vi "XP2i_Check_Error.vi"(4 "Error Code":T6=5490, 6 "Driver Name":T7="B1_28", 8 "Error In":errorcluster, 11 "DriverConnect in":T1={"InterfaceType"=enum."VISA", "OpenedSession"="COM4", "InterfaceSettings"={"Interface"=enum."RS232", "EOS 4 read"=enum."Default (=EOS 4 write)", "EOS 4 write"=enum."CR (\\r)", "TMO, ms"=2000, "Sett"=variant(cluster{"Baud Rate":u32, "Data Bits":u16, "Parity":u16, "Stop Bits":u16, "Flow Control":u16, "Eho":bool} {"Baud Rate"=75, "Data Bits"=0, "Parity"=0, "Stop Bits"=0, "Flow Control"=0, "Eho"=FALSE})}}) -> (0 "Error Out":errorcluster, 3 "DriverConnect out":T1={"InterfaceType"=enum."VISA", "OpenedSession"="COM4", "InterfaceSettings"={"Interface"=enum."RS232", "EOS 4 read"=enum."Default (=EOS 4 write)", "EOS 4 write"=enum."CR (\\r)", "TMO, ms"=2000, "Sett"=variant(cluster{"Baud Rate":u32, "Data Bits":u16, "Parity":u16, "Stop Bits":u16, "Flow Control":u16, "Eho":bool} {"Baud Rate"=75, "Data Bits"=0, "Parity"=0, "Stop Bits"=0, "Flow Control"=0, "Eho"=FALSE})}})   [LabVIEW 2018]
uses:
  MOKO_LabViewLibrary/MokoLowLevel/MokoLowLovelControl/MLLC_DriverName.ctl
  MOKO_LabViewLibrary/MokoLowLevel/MokoLowLovelControl/MLLC_ErrorCode.ctl
  MOKO_LabViewLibrary/MokoLowLevel/MokoLowLovelControl/MLLC_ConnectCluster.ctl
  MOKO_LabViewLibrary/MokoLowLevel/MokoLowLovelControl/MLLC_InterfaceType.ctl
  MOKO_LabViewLibrary/MokoLowLevel/MokoLowLovelControl/MLLC_OpenedSession.ctl
  MOKO_LabViewLibrary/MokoLowLevel/MokoLowLovelControl/MLLC_InterfaceSettings.ctl
  MOKO_LabViewLibrary/MokoLowLevel/MokoLowLovelControl/MLLC_InterfaceKind.ctl
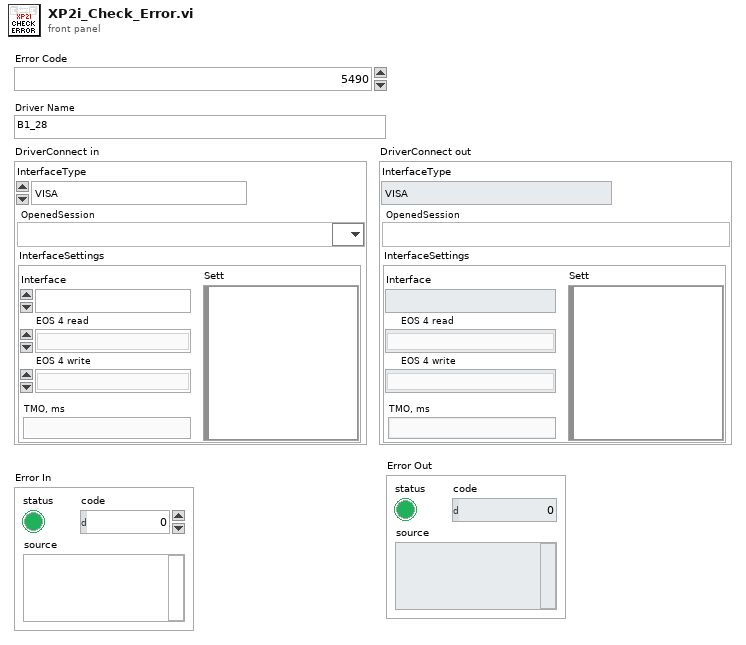
[diagram p1: front panel]
types:
  T1 = typedef "MLLC_ConnectCluster.ctl" = cluster{"InterfaceType":T2, "OpenedSession":T3, "InterfaceSettings":T4}
  T2 = typedef "MLLC_InterfaceType.ctl" = enum16{"VISA", "Prologix USB-GPIB"}
  T3 = typedef "MLLC_OpenedSession.ctl" = refnum<visa-resource-name>
  T4 = typedef "MLLC_InterfaceSettings.ctl" = cluster{"Interface":T5, "EOS 4 read":enum16{"Default (=EOS 4 write)", "CR (\\r)", "LF (\\n)", "None"}, "EOS 4 write":enum16{"CR+LF (\\r\\n)", "CR (\\r)", "LF (\\n)", "None"}, "TMO, ms":i32, "Sett":variant}
  T5 = typedef "MLLC_InterfaceKind.ctl" = enum16{"RS232", "GPIB", "USB", "Ethernet", "another"}
  T6 = typedef "MLLC_ErrorCode.ctl" = u32
  T7 = typedef "MLLC_DriverName.ctl" = string
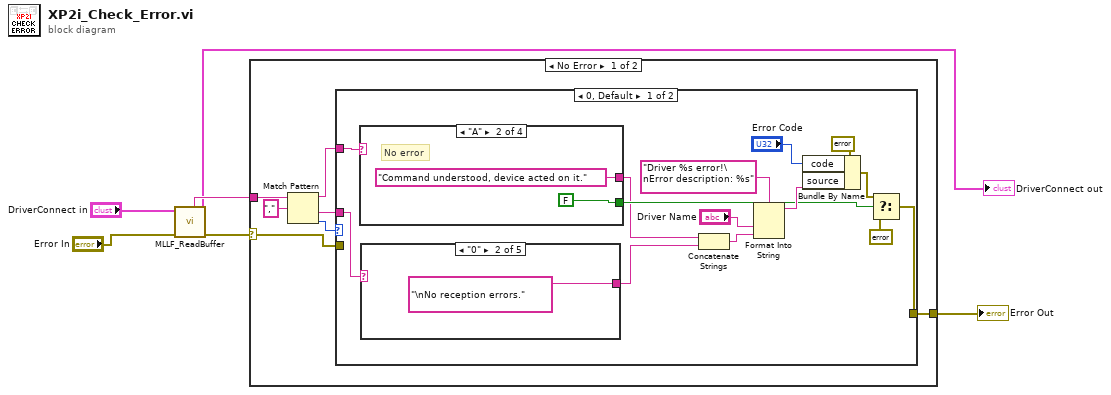
[diagram p0: block diagram]
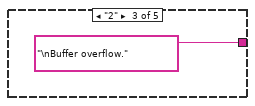
[diagram p3: hidden frame]
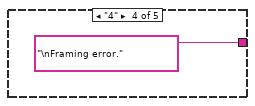
[diagram p4: hidden frame]
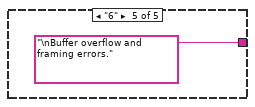
[diagram p5: hidden frame]
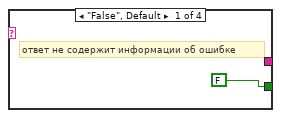
[diagram p6: hidden frame]
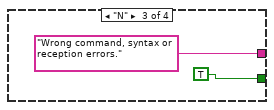
[diagram p7: hidden frame]
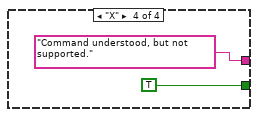
[diagram p8: hidden frame]
diagram:
  n1 = call "MLLF_ReadBuffer.vi"("Error In"="Error In", "DriverConnect in"="DriverConnect in") -> ("Error Out"=w5:errorcluster, "DriverConnect out"=→"DriverConnect out":T1, "String"=w6:string)  [unwired: 6 in]
  n2 = case shown="No Error" w5 {
    selector: w5 -> [w7 w40]
    tunnel: [w8 w40] -> w3
    tunnel: w6 -> [w13 _]
    frame No Error {
      n3 = Match Pattern(string=w13, regular expression=",") -> (before substring=w10:string, after substring=w9:string, offset past match=w11:i32)  [unwired: 1 in, 1 out]
      n4 = case shown="0, Default" w11 {
        tunnel: w10 -> [w27 _]
        tunnel: w9 -> [w17 _]
        tunnel: [w19 w39] -> w8
        tunnel: w7 -> [_ w39]
        frame 0, Default {
          n5 = case shown="\"A\"" w27 {
            tunnel: [FALSE ("s") FALSE ("s") TRUE ("s") TRUE ("s")] -> w18
            tunnel: [_ "Command understood, device acted on it." ("format string") "Wrong command, syntax or reception errors." ("format string") "Command understood, but not supported." ("format string")] -> w15
            frame "False", Default {
              # "ответ не содержит информации об ошибке"
            }
            frame "A" {
              # "No error"
            }
            frame "N" {
            }
            frame "X" {
            }
          }
          n6 = case shown="\"0\"" w17 {
            tunnel: [_ "\nNo reception errors." ("format string") "\nBuffer overflow." ("format string") "\nFraming error." ("format string") "\nBuffer overflow and framing errors." ("format string")] -> w14
            frame "False", Default {
              # "ответ не содержит информации \nо приеме команд"
            }
            frame "0" {
            }
            frame "2" {
            }
            frame "4" {
            }
            frame "6" {
            }
          }
          n7 = Concatenate Strings(w15, w14) -> (w16:string)
          n8 = Format Into String(format string="Driver %s error!\nError description: %s", "Driver Name", w16) -> (resulting string=w24:string)  [unwired: 2 in, 1 out]
          n9 = Bundle By Name(cluster=errorcluster {"status"=TRUE, "code"=0, "source"=""} ("error in"), "code"="Error Code", "source"=w24) -> (w21:errorcluster)
          n10 = Select(t=w21, s=w18, f=errorcluster {"status"=FALSE, "code"=0, "source"=""}) -> (s? t:f=w19:errorcluster)
        }
        frame -1 {
          # "как обрабатывать в этом случае?"
          # "запятая не найдена, значит этот ответ не содержит информации об ошибке"
        }
      }
    }
    frame Error {
    }
  }
  "Error Out" <- w3
